vi "ABR-Plot Traces.vi"(0 "Analysis":T1, 1 "Avg Mode":enum16{"Neural/CM", "ANOW"}(ring), 9 "Normalize individual?":bool, 11 "error in (no error)":errorcluster, 12 "Neural Ref":refnum<vi>, 13 "CM Ref":refnum<vi>) -> (15 "error out":errorcluster)   [LabVIEW 2020]
uses:
  Typedefs/ABR-Analysis State.ctl
  Threshold Estimation VIs/ABR3-Threshold Estimation Result.ctl
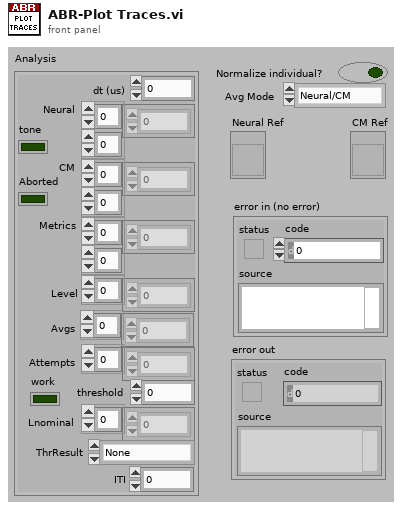
[diagram p1: front panel]
types:
  T1 = typedef "ABR-Analysis State.ctl" = cluster{"dt (us)":dbl, "Neural":dbl[][], "CM":dbl[][], "Metrics":dbl[][], "Level":dbl[], "Avgs":i32[], "Attempts":i32[], "Aborted":bool, "threshold":dbl, "Lnominal":dbl[], "tone":bool, "work":bool, "ThrResult":T2, "ITI":dbl}
  T2 = typedef "ABR3-Threshold Estimation Result.ctl" = enum16{"None", "Power", "Sigmoid", "Power (noisy)", "Suprathreshold", "Invalid"}
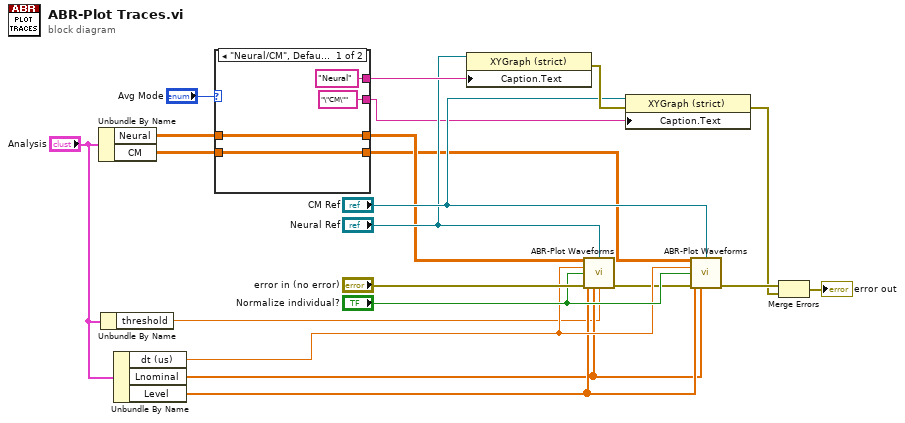
[diagram p0: block diagram]
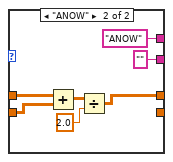
[diagram p2: hidden frame]
diagram:
  n1 = Unbundle By Name("Analysis") -> ("Neural"=w8:dbl[][], "CM"=w7:dbl[][])
  n2 = Unbundle By Name("Analysis") -> ("threshold"=w2:dbl)
  n3 = Unbundle By Name("Analysis") -> ("dt (us)"=w19:dbl, "Lnominal"=w4:dbl[], "Level"=w17:dbl[])
  n4 = case shown="\"Neural/CM\", Default" "Avg Mode" {
    tunnel: ["Neural" ("Plot.Plot Name") "ANOW" ("Plot.Plot Name")] -> w15
    tunnel: ["\"CM\"" ("Plot.Plot Name") "" ("Plot.Plot Name")] -> w11
    tunnel: w8 -> [w23 w30]
    tunnel: w7 -> [w22 w29]
    tunnel: [w23 w26] -> w6
    tunnel: [w22 _] -> w5
    frame "Neural/CM", Default {
    }
    frame "ANOW" {
      n5 = Add(x=w30, y=w29) -> (x+y=w28:dbl[][])
      n6 = Divide(x=w28, y=2.0) -> (x/y=w26:dbl[][])
    }
  }
  n7 = property class="XYGraph (strict)"(reference="Neural Ref", "Caption.Text"=w15) -> (error out=w14:errorcluster)  [unwired: 1 in, 1 out]
  n8 = call "ABR-Plot Waveforms.vi"("Array"=w6, "graph ref"="Neural Ref", "dt (us)"=w19, "Normalize traces"="Normalize individual?", "Seqvals"=w17, "error in (no error)"="error in (no error)", "InnerVals"=w4, "Threshold"=w2) -> ("error out"=w1:errorcluster)  [unwired: 7 in]
  n9 = property class="XYGraph (strict)"(reference="CM Ref", error in=w14, "Caption.Text"=w11) -> (error out=w9:errorcluster)  [unwired: 1 out]
  n10 = call "ABR-Plot Waveforms.vi"("Array"=w5, "graph ref"="CM Ref", "dt (us)"=w19, "Normalize traces"="Normalize individual?", "Seqvals"=w17, "error in (no error)"=w1, "InnerVals"=w4) -> ("error out"=w18:errorcluster)  [unwired: 8 in]
  n11 = Merge Errors(w18, w9) -> (→"error out":errorcluster)
